vi "Read AC Output.vi"(8 "error in (no error)":errorcluster, 11 "VISA resource name":refnum<visa-resource-name>) -> (0 "error out":errorcluster, 1 "Actual AC Current Level (A)":dbl format="%.4g", 2 "Actual AC Voltage Level (V)":dbl format="%.4g", 3 "VISA resource name out":refnum<visa-resource-name>, 4 "Output Frequency (Hz)":dbl format="%.4g")   [LabVIEW 2015, in "BK Precision 983X Series.lvlib"]
doc: "Returns the actual AC voltage level,actual AC current level, and the output frequency."
uses:
  <instrlib>/BK Precision 983X Series/BK Precision 983X Series.lvlib
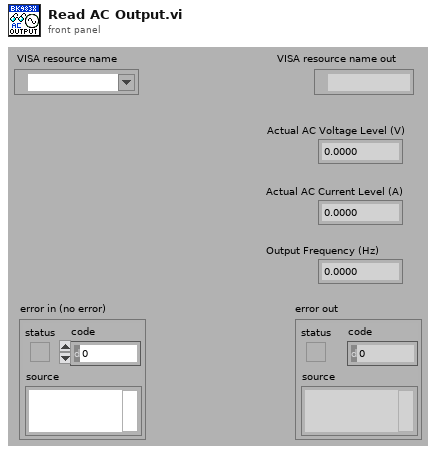
[diagram p1: front panel]
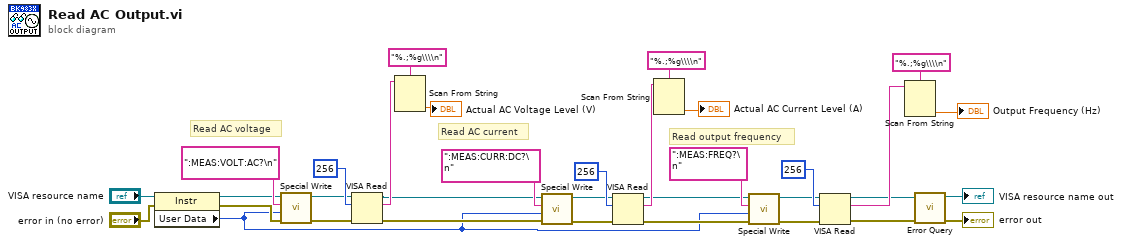
[diagram p0: block diagram]
diagram:
  # "Read output frequency"
  # "Read AC voltage"
  # "Read AC current"
  n1 = property class="Instr"(reference="VISA resource name", error in="error in (no error)") -> (reference out=w23:refnum<visa-resource-name>, error out=w22:errorcluster, "User Data"=w5:u32)
  n2 = call <instrlib>:"Special Write.vi"("error in (no error)"=w22, "Delay (0 ms)"=w5, "Input String"=":MEAS:VOLT:AC?\n" ("format string"), "VISA resource name"=w23) -> ("error out"=w27:errorcluster, "VISA resource name out"=w28:refnum<visa-resource-name>)  [unwired: 6 in]
  n3 = VISA Read(VISA resource name=w28, byte count=u32 256, error in (no error)=w27) -> (VISA resource name out=w9:refnum<visa-resource-name>, read buffer=w31:string, error out=w8:errorcluster)  [unwired: 1 out]
  n4 = Scan From String(format string="%.;%g\\\\n", input string=w31) -> (output 1=→"Actual AC Voltage Level (V)":dbl)  [unwired: 3 in, 3 out]
  n5 = call <instrlib>:"Special Write.vi"("error in (no error)"=w8, "Delay (0 ms)"=w5, "Input String"=":MEAS:CURR:DC?\n" ("format string"), "VISA resource name"=w9) -> ("error out"=w17:errorcluster, "VISA resource name out"=w18:refnum<visa-resource-name>)  [unwired: 6 in]
  n6 = VISA Read(VISA resource name=w18, byte count=u32 256, error in (no error)=w17) -> (VISA resource name out=w7:refnum<visa-resource-name>, read buffer=w20:string, error out=w6:errorcluster)  [unwired: 1 out]
  n7 = Scan From String(format string="%.;%g\\\\n", input string=w20) -> (output 1=→"Actual AC Current Level (A)":dbl)  [unwired: 3 in, 3 out]
  n8 = call <instrlib>:"Special Write.vi"("error in (no error)"=w6, "Delay (0 ms)"=w5, "Input String"=":MEAS:FREQ?\n" ("format string"), "VISA resource name"=w7) -> ("error out"=w11:errorcluster, "VISA resource name out"=w12:refnum<visa-resource-name>)  [unwired: 6 in]
  n9 = VISA Read(VISA resource name=w12, byte count=u32 256, error in (no error)=w11) -> (VISA resource name out=w2:refnum<visa-resource-name>, read buffer=w14:string, error out=w1:errorcluster)  [unwired: 1 out]
  n10 = Scan From String(format string="%.;%g\\\\n", input string=w14) -> (output 1=→"Output Frequency (Hz)":dbl)  [unwired: 3 in, 3 out]
  n11 = call <instrlib>:"Error Query.vi"("error in (no error)"=w1, "VISA resource name"=w2) -> ("error out"=→"error out":errorcluster, "VISA resource name out"=→"VISA resource name out":refnum<visa-resource-name>)  [unwired: 6 in, 2 out]
